vi "write camera json.vi"(8 "error in (no error)":errorcluster, 11 "Save Image in":refnum<class "Save Image.lvclass">) -> (0 "error out":errorcluster, 3 "Save Image out":refnum<class "Save Image.lvclass">)   [LabVIEW 2018, in "Save Image.lvclass"]
doc: "Prepare the header content to be provided to the Python toolkit\n\nThis function returns a JSON with the information to be written into the image header"
uses:
  Save Image.lvclass
  Save Image.lvclass/Save Image.ctl
  Channel/Channel.lvclass/Channel.ctl
  Simulated_CCD_Camera/Simulated Camera.lvclass
  Channel/Channel.lvclass
panel:
  out "timmings":T1
  out "prev SET parameters":T2
  out "CCD Config":T3
  out "Camera Status":T4
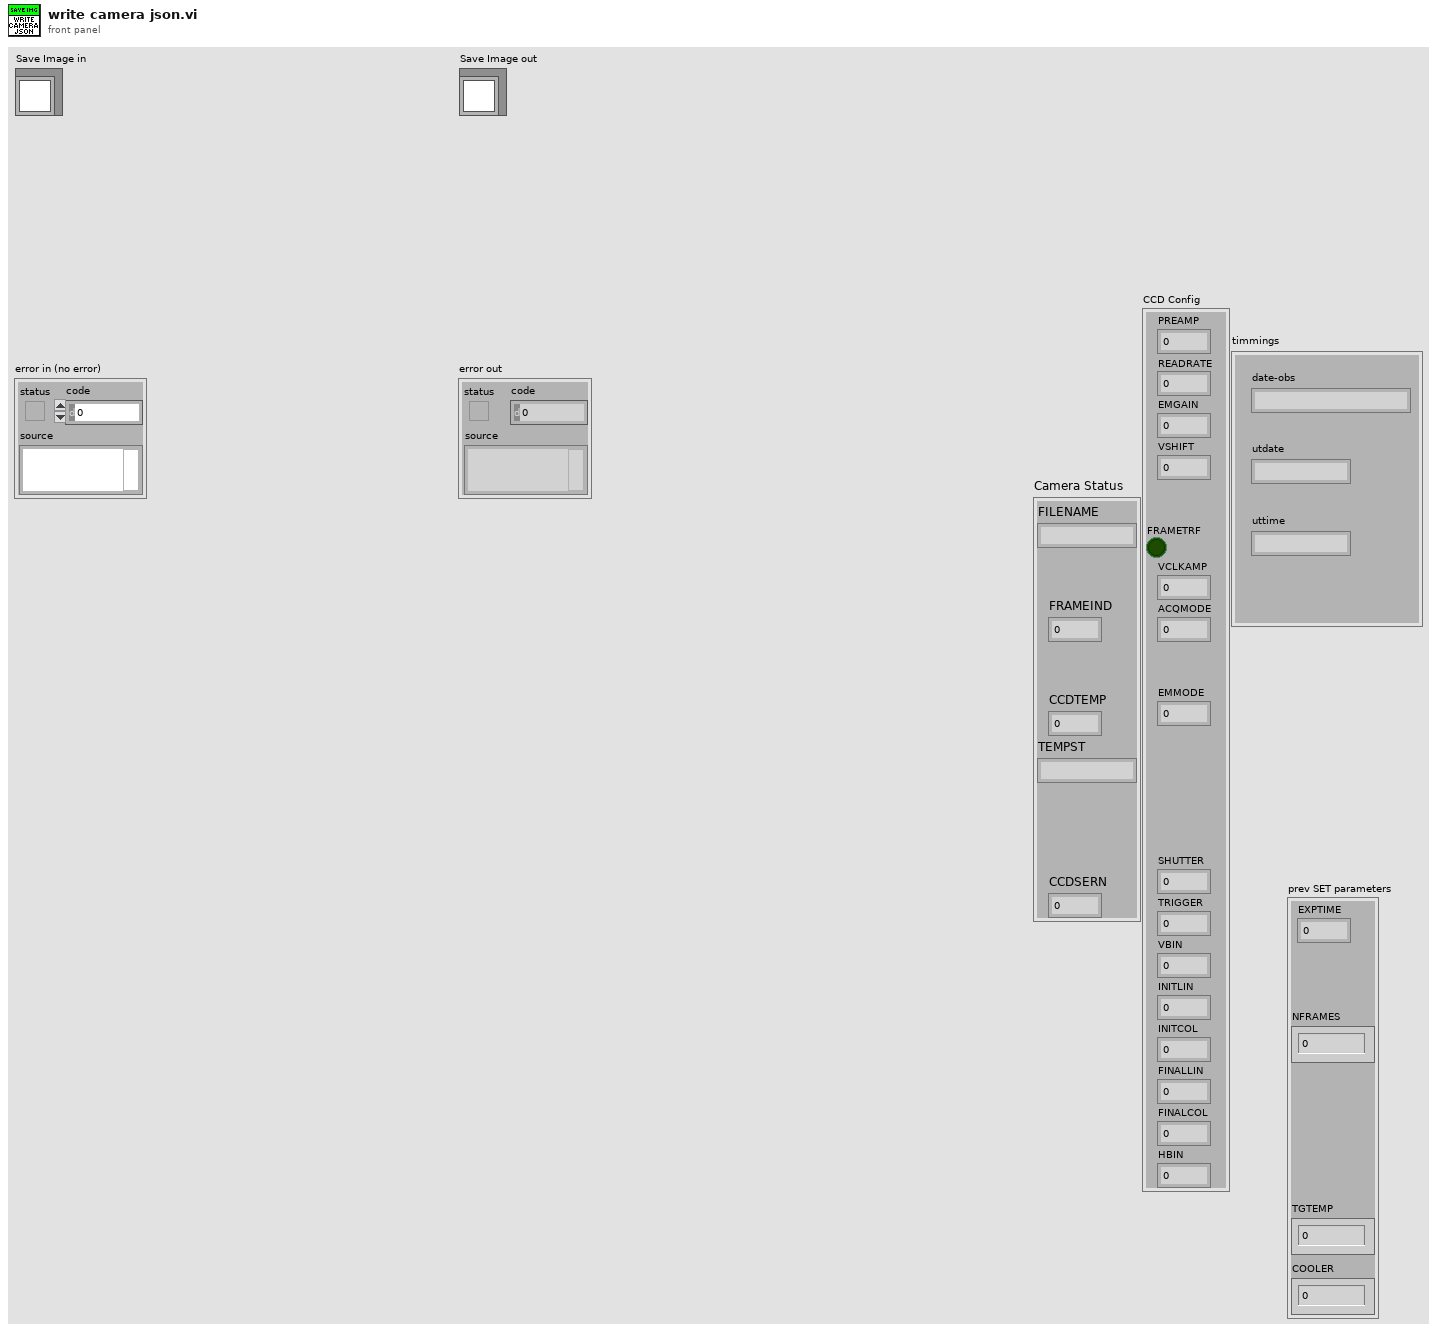
[diagram p1: front panel]
types:
  T1 = cluster{"date-obs":string, "utdate":string, "uttime":string}
  T2 = cluster{"EXPTIME":sgl, "NFRAMES":u32, "TGTEMP":i32, "COOLER":u16}
  T3 = cluster{"PREAMP":u16, "READRATE":u16, "EMGAIN":u16, "VSHIFT":u16, "FRAMETRF":bool, "VCLKAMP":u16, "ACQMODE":u16, "EMMODE":u16, "SHUTTER":u16, "TRIGGER":u16, "VBIN":u16, "INITLIN":u16, "INITCOL":u16, "FINALLIN":u16, "FINALCOL":u16, "HBIN":u16}
  T4 = cluster{"FILENAME":string, "FRAMEIND":u16, "CCDTEMP":i16, "TEMPST":string, "CCDSERN":u16}
  T5 = cluster{"CYCLES_DONE":u16, "LAST_IMAGE_NAME":string, "USED_DISK_SPACE":u16, "FRAMES_DONE":u16, "CCD_STATUS":string, "CURRENT_TEMPERATURE":i16, "TEMPERATURE_STATUS":string, "FRAME_EXPOSURE_TIME":sgl, "ERROR":bool, "SERIAL_NUMBER":u16, "ACQUIRING":bool, "IMAGE_INDEX":u32, "SEQS_DONE":u16}
  T6 = cluster{"PREAMP":u16, "READOUT_RATE":u16, "EM_GAIN":u16, "VERTICAL_SHIFT_SPEED":u16, "READ_MODE":u16, "FRAME_TRANSFER":bool, "VERTICAL_CLOCK_VOLTAGE":u16, "ACQUISITION_MODE":u16, "AD_CHANNEL":u16, "EM_MODE":u16, "SHUTTER_TTL":u16, "SHUTTER_OPENING_TIME":u16, "SHUTTER_CLOSING_TIME":u16, "SHUTTER_MODE":u16, "TRIGGER_MODE":u16, "VBIN":u16, "INITIAL_LINE":u16, "INITIAL_COLUMN":u16, "FINAL_LINE":u16, "FINAL_COLUMN":u16, "HBIN":u16}
  T7 = cluster{"COOLER_POWER_STATUS":u16, "TEMP":i32, "EXPTIME":dbl, "#FRAMES":u32}
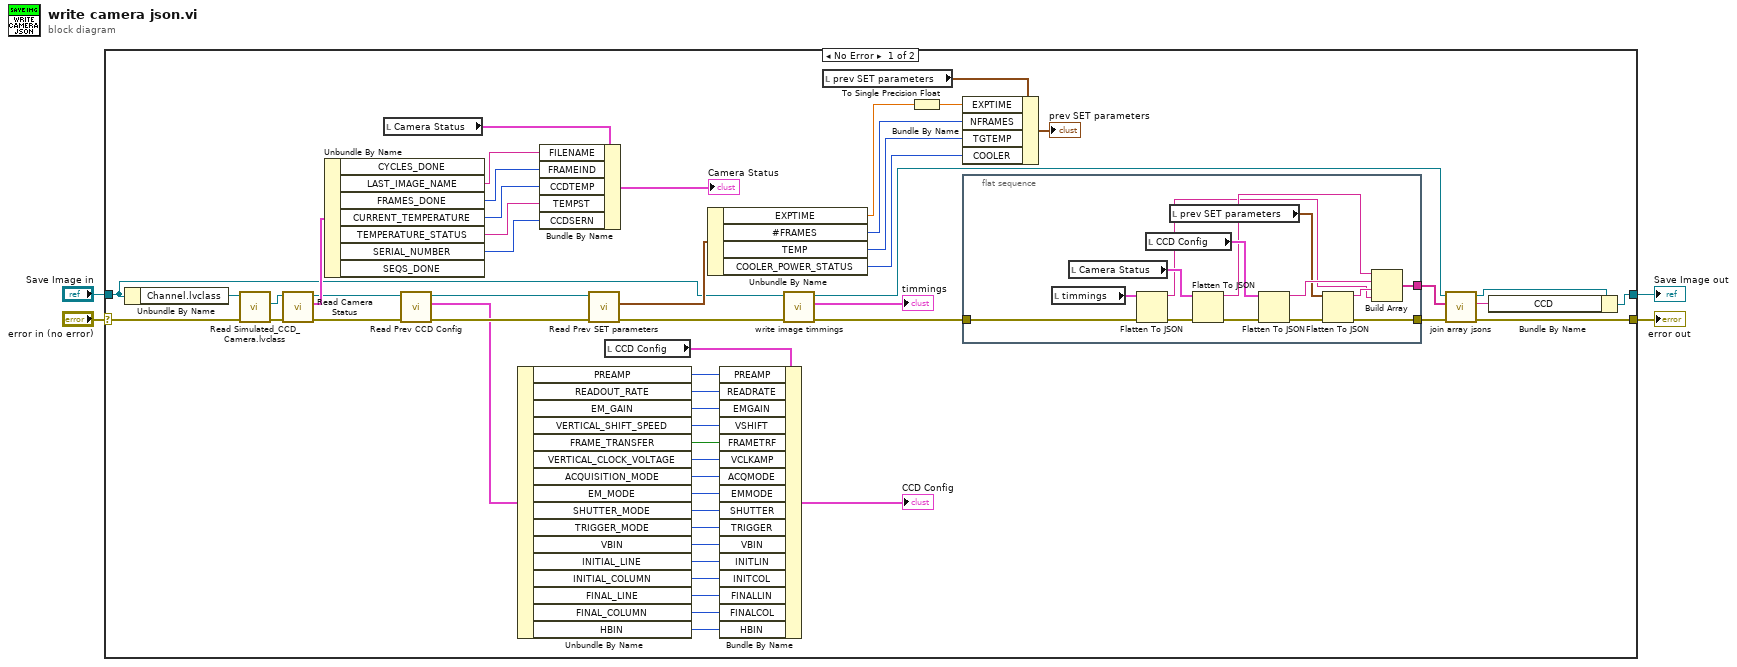
[diagram p0: block diagram]
diagram:
  n1 = case shown="No Error" "error in (no error)" {
    selector: "error in (no error)" -> [w19 w74]
    tunnel: [w5 w74] -> w3
    tunnel: [w7 w73] -> w1
    tunnel: "Save Image in" -> [w13 w73]
    frame No Error {
      n2 = Unbundle By Name(w13) -> ("Channel.lvclass"=w20:refnum<class "Channel.lvclass">)
      n3 = call "Read Simulated_CCD_Camera.lvclass.vi"("error in (no error)"=w19, "Channel in"=w20) -> ("error out"=w57:errorcluster, "Simulated_CCD_Camera.lvclass"=w58:refnum<class "Simulated Camera.lvclass">)  [unwired: 7 in, 1 out]
      n4 = call "Read Camera Status.vi"("error in (no error)"=w57, "CCDCamera in"=w58) -> ("error out"=w25:errorcluster, "Camera Status"=w52:T5, "CCDCamera out"=w24:refnum<class "Simulated Camera.lvclass">)  [unwired: 7 in]
      n5 = Unbundle By Name(w52) -> ("LAST_IMAGE_NAME"=w50:string, "FRAMES_DONE"=w49:u16, "CURRENT_TEMPERATURE"=w48:i16, "TEMPERATURE_STATUS"=w47:string, "SERIAL_NUMBER"=w51:u16)  [unwired: 2 out]
      n6 = local read "Camera Status"() -> (w53:T4)
      n7 = call-dynamic "Read Prev CCD Config.vi"("error in (no error)"=w25, "Simulated_CCD_Camera in"=w24) -> ("error out"=w55:errorcluster, "Prev CCD Config"=w44:T6, "Simulated_CCD_Camera out"=w56:refnum<class "Simulated Camera.lvclass">)  [unwired: 7 in]
      n8 = Unbundle By Name(w44) -> ("PREAMP"=w43:u16, "READOUT_RATE"=w42:u16, "EM_GAIN"=w41:u16, "VERTICAL_SHIFT_SPEED"=w40:u16, "FRAME_TRANSFER"=w39:bool, "VERTICAL_CLOCK_VOLTAGE"=w38:u16, "ACQUISITION_MODE"=w37:u16, "EM_MODE"=w36:u16, "SHUTTER_MODE"=w35:u16, "TRIGGER_MODE"=w34:u16, "VBIN"=w33:u16, "INITIAL_LINE"=w32:u16, "INITIAL_COLUMN"=w31:u16, "FINAL_LINE"=w30:u16, "FINAL_COLUMN"=w29:u16, "HBIN"=w28:u16)
      n9 = Bundle By Name(cluster=w53, "FILENAME"=w50, "FRAMEIND"=w49, "CCDTEMP"=w48, "TEMPST"=w47, "CCDSERN"=w51) -> (→"Camera Status":T4)
      n10 = call-dynamic "Read Prev SET parameters.vi"("error in (no error)"=w55, "Simulated_CCD_Camera in"=w56) -> ("error out"=w15:errorcluster, "Prev SET parameters"=w27:T7)  [unwired: 7 in, 1 out]
      n11 = local read "CCD Config"() -> (w45:T3)
      n12 = Unbundle By Name(w27) -> ("EXPTIME"=w22:dbl, "#FRAMES"=w18:u32, "TEMP"=w17:i32, "COOLER_POWER_STATUS"=w16:u16)
      n13 = Bundle By Name(cluster=w45, "PREAMP"=w43, "READRATE"=w42, "EMGAIN"=w41, "VSHIFT"=w40, "FRAMETRF"=w39, "VCLKAMP"=w38, "ACQMODE"=w37, "EMMODE"=w36, "SHUTTER"=w35, "TRIGGER"=w34, "VBIN"=w33, "INITLIN"=w32, "INITCOL"=w31, "FINALLIN"=w30, "FINALCOL"=w29, "HBIN"=w28) -> (→"CCD Config":T3)
      n14 = call "write image timmings.vi"("error in (no error)"=w15, "Save Image in"=w13) -> ("error out"=w14:errorcluster, "timmings"=→"timmings":T1, "Save Image out"=w9:refnum<class "Save Image.lvclass">)  [unwired: 7 in]
      n15 = local read "prev SET parameters"() -> (w26:T2)
      n16 = To Single Precision Float(number=w22) -> (single precision float=w21:sgl)
      n17 = Bundle By Name(cluster=w26, "EXPTIME"=w21, "NFRAMES"=w18, "TGTEMP"=w17, "COOLER"=w16) -> (→"prev SET parameters":T2)
      n18 = flat-sequence {
        tunnel: [w65] -> w10
        tunnel: [w66] -> w11
        tunnel: w14 -> [w62]
        frame #0 {
          n19 = local read "timmings"() -> (w60:T1)
          n20 = local read "Camera Status"() -> (w72:T4)
          n21 = Flatten To JSON(anything=w60, error in (no error)=w62) -> (JSON string=w59:string, 11:w61:errorcluster)  [unwired: 1 in]
          n22 = local read "CCD Config"() -> (w71:T3)
          n23 = local read "prev SET parameters"() -> (w64:T2)
          n24 = Flatten To JSON(anything=w72, error in (no error)=w61) -> (JSON string=w63:string, 11:w68:errorcluster)  [unwired: 1 in]
          n25 = Flatten To JSON(anything=w71, error in (no error)=w68) -> (JSON string=w70:string, 11:w67:errorcluster)  [unwired: 1 in]
          n26 = Flatten To JSON(anything=w64, error in (no error)=w67) -> (JSON string=w69:string, 11:w65:errorcluster)  [unwired: 1 in]
          n27 = Build Array(w63, w70, w69, w59) -> (w66:string[])
        }
      }
      n28 = call "join array jsons.vi"("error in (no error)"=w10, "jsons"=w11, "Save Image in"=w9) -> ("error out"=w5:errorcluster, "concatenated json"=w6:string, "Save Image out"=w8:refnum<class "Save Image.lvclass">)  [unwired: 6 in]
      n29 = Bundle By Name(cluster=w8, "CCD"=w6) -> (w7:refnum<class "Save Image.lvclass">)
    }
    frame Error {
    }
  }
  "error out" <- w3
  "Save Image out" <- w1
